vi "Read Tool Type from Tool.vi"(8 "error in (no error)":errorcluster) -> (0 "error out":errorcluster, 1 "Success":bool, 2 "Tool Type":u16, 3 "Message Data":variant, 5 "Data Count":i32)   [LabVIEW 2015, in "Tool Module.lvlib"]
uses:
  Tool Module.lvlib
  Tool Interface/Tool Interface.lvlib
panel:
  out "Data String Out":string
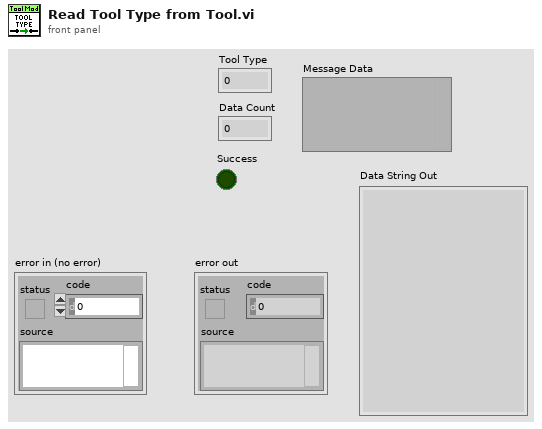
[diagram p1: front panel]
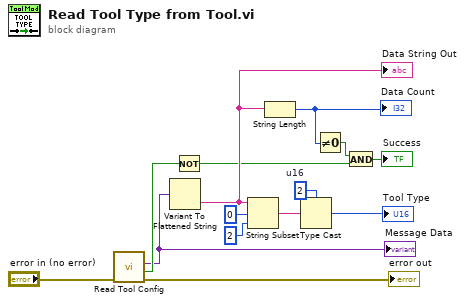
[diagram p0: block diagram]
diagram:
  w11 = u16 2  # u16
  n1 = call "Read Tool Config.vi"("error in (no error)"="error in (no error)") -> ("error out"=→"error out":errorcluster, "timed out?"=w5:bool, "Message Data"=w4:variant)  [unwired: 7 in, 1 out]
  "Message Data" <- w4
  n2 = Variant To Flattened String(Variant=w4) -> (data string=w6:string)  [unwired: 1 out]
  "Data String Out" <- w6
  n3 = Not(x=w5) -> (.not. x?=w1:bool)
  n4 = String Subset(string=w6, offset (0)=0, length (rest)=2 ("length (rest)")) -> (substring=w14:string)
  n5 = String Length(string=w6) -> (length=w7:i32)
  "Data Count" <- w7
  n6 = Type Cast(type=w11, x=w14) -> (*(type *) &x=→"Tool Type":u16)
  n7 = Not Equal To 0?(x=w7) -> (x != 0?=w9:bool)
  n8 = And(x=w9, y=w1) -> (x .and. y?=→"Success":bool)
